vi "PCRSize.vi"(0 "input cluster":T1={"Core"={"Current VI Reference"=refnum, "Close Panel on Exit?"=FALSE}, "Image Out"=refnum, "State"=0, "Points"={"Top Left"={"X"=0.0, "Y"=0.0}, "Top Right"={"X"=0.0, "Y"=0.0}, "Bottom Left"={"X"=0.0, "Y"=0.0}, "Bottom Right"={"X"=0.0, "Y"=0.0}, "x space 2"=0.0, "y space 2"=0.0, "x_space"=0.0, "y_space"=0.0, "Pixels"=[], "Fixpoint"={"X"=0.0, "Y"=0.0}}, "img_array"=[], "Temps"=[], "Temps_Array"=[], "Scan Area"=0.0, "Fixpoint Area"=0.0, "Config"={"Freezing"={"Cutoff"=2.0, "EndIndex"=2}}, "PCR Size"=0, "ImageCount"=0, "ShowGradient"=FALSE, "Save Well data"=FALSE, "Save Blackbody data"=FALSE, "Save Temps For Offset"=FALSE} {"Points"."Bottom Right"."Y" format="%.2f"; "Points"."Bottom Right"."X" format="%.2f"; "Points"."Top Left"."Y" format="%.2f"; "Points"."Top Left"."X" format="%.2f"; "Points"."Top Right"."Y" format="%.2f"; "Points"."Top Right"."X" format="%.2f"; "Points"."Bottom Left"."Y" format="%.2f"; "Points"."Bottom Left"."X" format="%.2f"; "Points"."Fixpoint"."Y" format="%.2f"; "Points"."Fixpoint"."X" format="%.2f"}) -> (1 "Width":i32, 2 "Height":i32)   [LabVIEW 2024]
uses:
  DataCluster_TCAL.ctl
  <vilib>/vision/Image Controls.llb/IMAQ Image.ctl
  TCE_Config.ctl
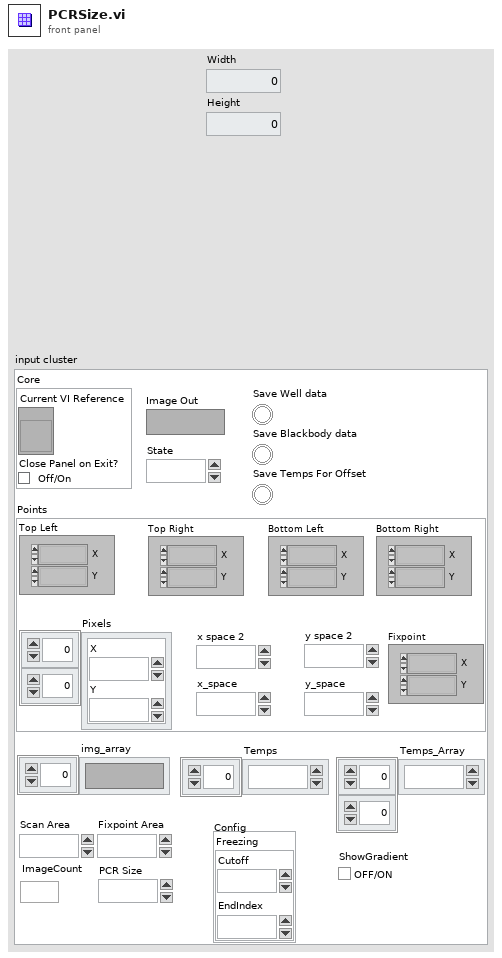
[diagram p1: front panel]
types:
  T1 = typedef "DataCluster_TCAL.ctl" = cluster{"Core":cluster{"Current VI Reference":refnum<vi>, "Close Panel on Exit?":bool}, "Image Out":T2, "State":i32, "Points":cluster{"Top Left":T3, "Top Right":T3, "Bottom Left":T3, "Bottom Right":T3, "x space 2":dbl, "y space 2":sgl, "x_space":sgl, "y_space":sgl, "Pixels":cluster{"X":i32, "Y":i32}[][], "Fixpoint":T3}, "img_array":T2[], "Temps":dbl[], "Temps_Array":dbl[][], "Scan Area":dbl, "Fixpoint Area":dbl, "Config":T4, "PCR Size":u16, "ImageCount":i32, "ShowGradient":bool, "Save Well data":bool, "Save Blackbody data":bool, "Save Temps For Offset":bool}
  T2 = typedef "IMAQ Image.ctl" = refnum<image>
  T3 = typedef "IMAQ Point" = cluster{"X":sgl, "Y":sgl}
  T4 = typedef "TCE_Config.ctl" = cluster{"Freezing":cluster{"Cutoff":dbl, "EndIndex":i32}}
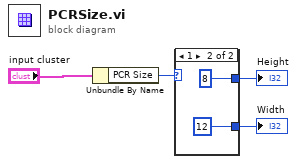
[diagram p0: block diagram]
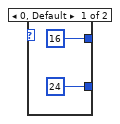
[diagram p2: hidden frame]
diagram:
  n1 = Unbundle By Name("input cluster") -> ("PCR Size"=w4:u16)
  n2 = case shown="1" w4 {
    tunnel: [24 12] -> w3
    tunnel: [16 8] -> w2
    frame 0, Default {
    }
    frame 1 {
    }
  }
  "Width" <- w3
  "Height" <- w2
